vi "AlliGator Read PI Imaging File Metadata.vi"(8 "error in":errorcluster, 11 "Image Folder":path) -> (0 "error out":errorcluster, 1 "Metadata":T1 {"Date" format="%<%x %.3X>T"}, 3 "Metadata String":string, 4 "bitness":i32, 6 "Correct bit shift":bool)   [LabVIEW 2021, in "AlliGator Files.lvlib"]
doc: "Extracts & decodes all metadata from a Pi Imaging gate image file."
uses:
  AlliGator Files.lvlib
  AlliGator RecSettings Metadata.ctl
  <vilib>/Utility/error.llb/Error Cluster From Error Code.vi
  <vilib>/ErrorRing/Error Ring.xnode
  Files/Files.lvlib
panel:
  # "see the AlliGator License on the block diagram (Ctrl+E or Window:Show Block Diagram)"
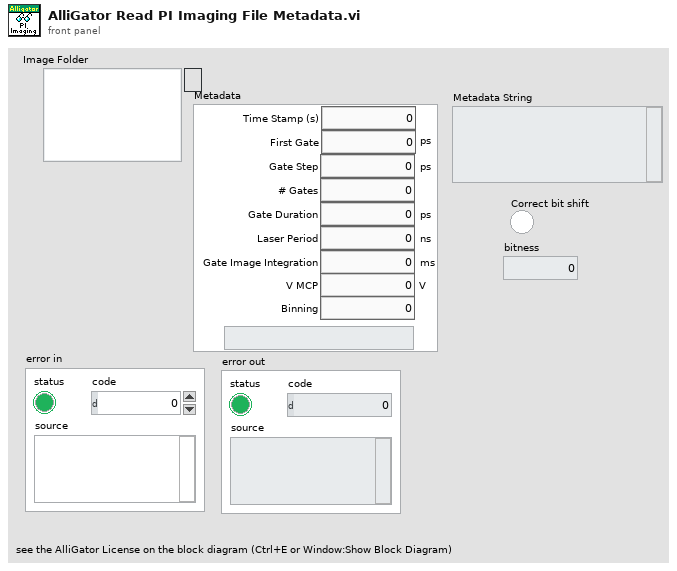
[diagram p1: front panel]
types:
  T1 = typedef "AlliGator Files.lvlib/AlliGator RecSettings Metadata.ctl" = cluster{"Time Stamp (s)":dbl, "First Gate":dbl[unit], "Gate Step":dbl[unit], "# Gates":i32, "Gate Duration":dbl[unit], "Laser Period":dbl[unit], "Gate Image Integration":dbl[unit], "Date":timestamp, "V MCP":dbl[unit], "Binning":dbl}
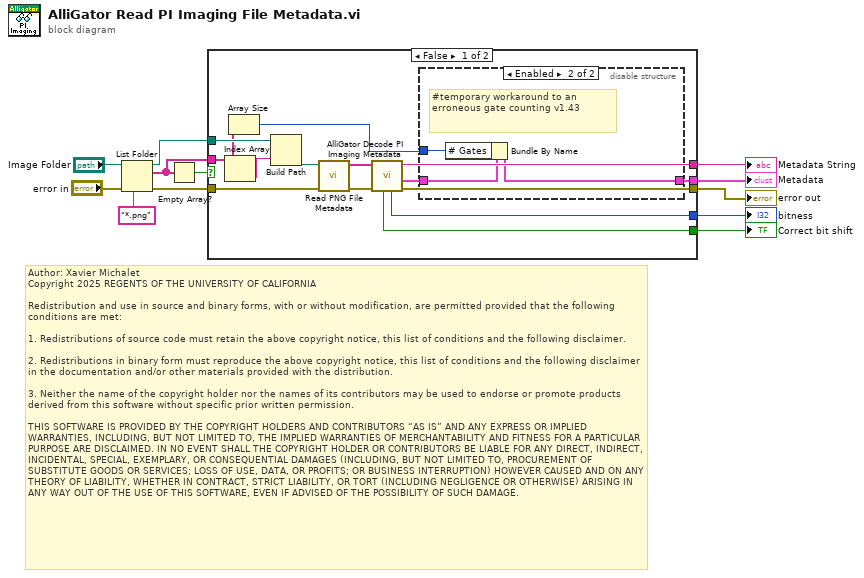
[diagram p0: block diagram]
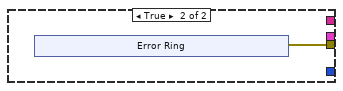
[diagram p3: hidden frame]
diagram:
  # "Author: Xavier Michalet\nCopyright 2025 REGENTS OF THE UNIVERSITY OF CALIFORNIA\n\nRedistribution and use in source and binary forms, with or without modification, are permitted provided that the following conditions are met:\n\n1. Redistributions of source code must retain the above copyright notice, this list of conditions and the following disclaimer.\n\n2. Redistributions in binary form must reproduce the above copyright notice, this list of conditions and the following disclaimer in the documentation and/or other materials provided with the distribution.\n\n3. Neither the name of the copyright holder nor the names of its contributors may be used to endorse or promote products derived from this software without specific prior written permission.\n\nTHIS SOFTWARE IS PROVIDED BY THE COPYRIGHT HOLDERS AND CONTRIBUTORS “AS IS” AND ANY EXPRESS OR IMPLIED WARRANTIES, INCLUDING, BUT NOT LIMITED TO, THE IMPLIED WARRANTIES OF MERCHANTABILITY AND FITNESS FOR A PARTICULAR PURPOSE ARE DISCLAIMED. IN NO EVENT SHALL THE COPYRIGHT HOLDER OR CONTRIBUTORS BE LIABLE FOR ANY DIRECT, INDIRECT, INCIDENTAL, SPECIAL, EXEMPLARY, OR CONSEQUENTIAL DAMAGES (INCLUDING, BUT NOT LIMITED TO, PROCUREMENT OF SUBSTITUTE GOODS OR SERVICES; LOSS OF USE, DATA, OR PROFITS; OR BUSINESS INTERRUPTION) HOWEVER CAUSED AND ON ANY THEORY OF LIABILITY, WHETHER IN CONTRACT, STRICT LIABILITY, OR TORT (INCLUDING NEGLIGENCE OR OTHERWISE) ARISING IN ANY WAY OUT OF THE USE OF THIS SOFTWARE, EVEN IF ADVISED OF THE POSSIBILITY OF SUCH DAMAGE."
  n1 = List Folder(path="Image Folder", pattern="*.png", error in="error in") -> (path out=w7:path, filenames=w6:string[], error out=w9:errorcluster)  [unwired: 1 in, 1 out]
  n2 = Empty Array?(array=w6) -> (empty?=w8:bool)
  n3 = case shown="False" w8 {
    tunnel: w9 -> [w23 _]
    tunnel: w7 -> [w26 _]
    tunnel: w6 -> [w16 _]
    tunnel: [w20 _] -> w5
    tunnel: [w17 _] -> w4
    tunnel: [w19 w31] -> w3
    tunnel: [w14 _] -> w2
    tunnel: [w13 _] -> w1
    frame False {
      n4 = Index Array(array=w16) -> (element=w25:string)  [unwired: 1 in]
      n5 = Array Size(array=w16) -> (size(s)=w15:i32)
      n6 = Build Path(base path=w26, name or relative path=w25) -> (appended path=w24:path)
      n7 = call "Read PNG File Metadata.vi"("Error In"=w23, "File Path"=w24) -> ("Error Out"=w22:errorcluster, "Metadata Text Fields"=w21:string[])  [unwired: 7 in, 1 out]
      n8 = call "AlliGator Decode PI Imaging Metadata.vi"("Error In"=w22, "Metadata Text Fields"=w21) -> ("Error Out"=w19:errorcluster, "Metadata"=w18:T1, "Metadata String"=w20:string, "bitness"=w13:i32, "Correct bit shift"=w14:bool)  [unwired: 5 in]
      n9 = disable-structure shown="Enabled" {
        disable-tunnel: w18 -> [w27 w30]
        disable-tunnel: [w27 w29] -> w17
        disable-tunnel: w15 -> [_ w28]
        frame Disabled {
        }
        frame Enabled {
          # "#temporary workaround to an erroneous gate counting v1.43"
          n10 = Bundle By Name(cluster=w30, "# Gates"=w28) -> (w29:T1)
        }
      }
    }
    frame True {
      n11 = xnode "Error Ring"() -> ("error out"=w31:errorcluster)
    }
  }
  "Metadata" <- w4
  "error out" <- w3
  "Metadata String" <- w5
  "Correct bit shift" <- w2
  "bitness" <- w1
